vi "Smart.vi"(2 "Power":dbl, 3 "Elevator Request":dbl) -> (0 "Encoder Distance from Top":dbl, 1 "Evevator motors power":dbl)   [LabVIEW 2014]
uses:
  Robot Global Data.vi
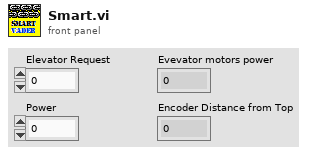
[diagram p1: front panel]
types:
  T1 = typedef "WPI_MotorControlDeviceRef.ctl" = cluster{"DeviceStatus":errorcluster, "Type":T2, "PWM":cluster{"Controller":T3, "PWM Channel":T4, "DeadBand":T5}, "CAN":cluster{"Device Number":u8, "Control Mode":T6, "Semaphore":T7, "Max Vout":dbl, "TalonSRX Control Mode":T8}, "Invert":bool, "TransformRef":T9, "InvTransformRef":T9}
  T2 = typedef "WPI_MotorControlType.ctl" = enum16{"PWM", "CAN", "CANTalonSRX"}
  T3 = typedef "FPGA_TypedefDigitalModule.ctl" = enum16{"Controller 1"}
  T4 = typedef "FPGA_DIOPWMChannel.ctl" = enum8{"PWM 0", "PWM 1", "PWM 2", "PWM 3", "PWM 4", "PWM 5", "PWM 6", "PWM 7", "PWM 8", "PWM 9", "PWM MXP 0", "PWM MXP 1", "PWM MXP 2", "PWM MXP 3", "PWM MXP 4", "PWM MXP 5", "PWM MXP 6", "PWM MXP 7", "PWM MXP 8", "PWM MXP 9", "Invalid"}
  T5 = typedef "WPI_PWMDeadband.ctl" = cluster{"Name":string, "maxPositivePwm":i32, "minPositivePwm":i32, "centerPwm":i32, "maxNegativePwm":i32, "minNegativePwm":i32, "angularRange":u16}
  T6 = typedef "WPI_CANJaguar_ControlMode.ctl" = enum8{"Percent VBus", "Current", "Speed", "Position", "Voltage"}
  T7 = typedef "Semaphore RefNum" = refnum<k1>
  T8 = typedef "WPI_CANTalonSRX_APIControlMode.ctl" = enum8{"Percent VBus", "Speed", "Position", "Slave", "Unchanged / Invalid"}
  T9 = typedef "WPI_PWMTransform_ConPane.ctl" = refnum<vi>
  T10 = typedef "WPI_EncoderDevRef.ctl" = cluster{"DevStatus":errorcluster, "EncoderIndex":T11, "CounterIndex":T12, "DistancePerCount":dbl, "Decoding Type":T13}
  T11 = typedef "FPGA_EncoderIdx.ctl" = enum8{"Enc 0", "Enc 1", "Enc 2", "Enc 3", "Enc 4", "Enc 5", "Enc 6", "Enc 7", "Invalid"}
  T12 = typedef "FPGA_CounterCtrSystemIndex.ctl" = enum8{"Ctr 0", "Ctr 1", "Ctr 2", "Ctr 3", "Ctr 4", "Ctr 5", "Ctr 6", "Ctr 7", "Invalid"}
  T13 = typedef "WPI_EncoderType.ctl" = enum16{"1x", "2x", "4x"}
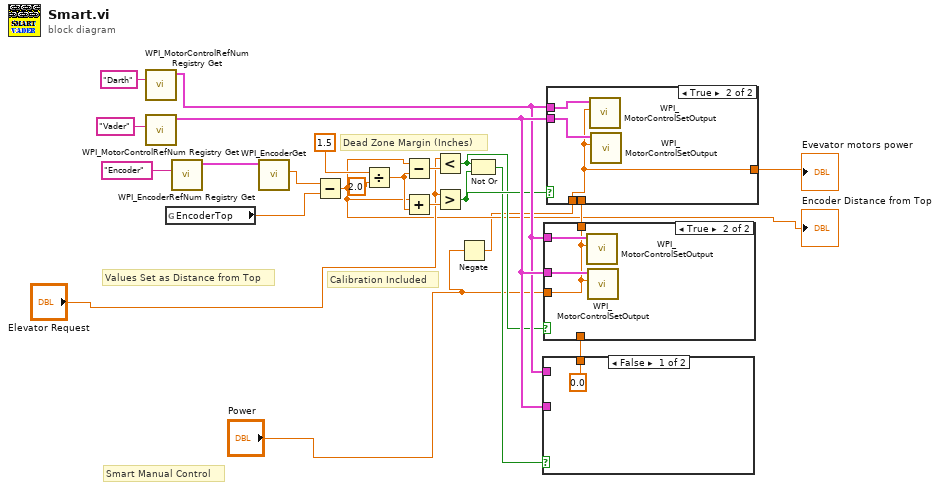
[diagram p0: block diagram]
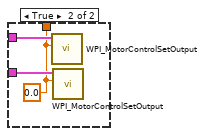
[diagram p2: hidden frame]
diagram:
  # "Dead Zone Margin (Inches)"
  # "Calibration Included"
  # "Values Set as Distance from Top"
  # "Smart Manual Control"
  n1 = call <vilib>:"WPI_MotorControlRefNum Registry Get.vi"("refnum name"="Darth") -> ("MotorControlDevRef"=w14:T1)  [unwired: 9 in, 1 out]
  n2 = call <vilib>:"WPI_MotorControlRefNum Registry Get.vi"("refnum name"="Vader") -> ("MotorControlDevRef"=w15:T1)  [unwired: 9 in, 1 out]
  n3 = global read "Robot Global Data.vi" "EncoderTop"() -> (w19:dbl)
  n4 = call <vilib>:"WPI_EncoderRefNum Registry Get.vi"("refnum name"="Encoder") -> ("EncoderDevRef"=w22:T10)  [unwired: 9 in, 1 out]
  n5 = call <vilib>:"WPI_EncoderGet.vi"("EncoderDevRef"=w22) -> ("Distance"=w18:dbl)  [unwired: 5 in, 5 out]
  n6 = Subtract(x=w18, y=w19) -> (x-y=w4:dbl)
  "Encoder Distance from Top" <- w4
  n7 = Divide(x=1.5 ("y"), y=2.0) -> (x/y=w8:dbl)
  n8 = Subtract(x=w4, y=w8) -> (x-y=w16:dbl)
  n9 = Add(x=w4, y=w8) -> (x+y=w17:dbl)
  n10 = Less?(x="Elevator Request", y=w16) -> (x < y?=w12:bool)
  n11 = Greater?(x="Elevator Request", y=w17) -> (0:w13:bool)
  n12 = Negate(x="Power") -> (-x=w2:dbl)
  n13 = Not Or(1:w13, 2:w12) -> (0:w11:bool)
  n14 = case shown="False" w11 {
    tunnel: w14 -> [_ w26]
    tunnel: w15 -> [_ w27]
    tunnel: [0.0 ("Output") w25] -> w6
    frame False {
    }
    frame True {
      w25 = 0.0 ("Output")
      n15 = call <vilib>:"WPI_MotorControlSetOutput.vi"("Output"=w25, "MotorControlDevRef"=w26) -> ()  [unwired: 7 in, 3 out]
      n16 = call <vilib>:"WPI_MotorControlSetOutput.vi"("Output"=w25, "MotorControlDevRef"=w27) -> ()  [unwired: 7 in, 3 out]
    }
  }
  n17 = case shown="True" w12 {
    tunnel: w14 -> [_ w31]
    tunnel: w15 -> [_ w30]
    tunnel: [w28 w29] -> w7
    tunnel: w6 -> [w28 _]
    tunnel: "Power" -> [_ w29]
    frame False {
    }
    frame True {
      n18 = call <vilib>:"WPI_MotorControlSetOutput.vi"("Output"=w29, "MotorControlDevRef"=w31) -> ()  [unwired: 7 in, 3 out]
      n19 = call <vilib>:"WPI_MotorControlSetOutput.vi"("Output"=w29, "MotorControlDevRef"=w30) -> ()  [unwired: 7 in, 3 out]
    }
  }
  n20 = case shown="True" w13 {
    tunnel: w14 -> [_ w35]
    tunnel: w15 -> [_ w34]
    tunnel: [w32 w33] -> w3
    tunnel: w7 -> [w32 _]
    tunnel: w2 -> [_ w33]
    frame False {
    }
    frame True {
      n21 = call <vilib>:"WPI_MotorControlSetOutput.vi"("Output"=w33, "MotorControlDevRef"=w35) -> ()  [unwired: 7 in, 3 out]
      n22 = call <vilib>:"WPI_MotorControlSetOutput.vi"("Output"=w33, "MotorControlDevRef"=w34) -> ()  [unwired: 7 in, 3 out]
    }
  }
  "Evevator motors power" <- w3
